vi "Gyro Angle.vi"() -> (13 "Angle":dbl)   [LabVIEW 2014]
uses:
  Global Variables/Refnum Names.vi
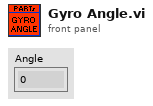
[diagram p1: front panel]
types:
  T1 = typedef "WPI_GyroDevRef.ctl" = cluster{"DevStatus":errorcluster, "Analog Module":T2, "Analog Channel":T3, "Offset":dbl, "Gain (VoltsPerDegree/Second)":dbl}
  T2 = typedef "FPGA_TypedefAnalogModule.ctl" = enum16{"Controller 1"}
  T3 = typedef "FPGA_AIChannel.ctl" = enum8{"AI 0", "AI 1", "AI 2", "AI 3", "AI MXP 0", "AI MXP 1", "AI MXP 2", "AI MXP 3", "Invalid"}
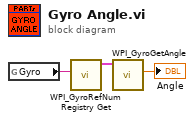
[diagram p0: block diagram]
diagram:
  n1 = global read "Refnum Names.vi" "Gyro"() -> (w2:string)
  n2 = call <vilib>:"WPI_GyroRefNum Registry Get.vi"("refnum name"=w2) -> ("GyroDevRef"=w1:T1)  [unwired: 9 in, 1 out]
  n3 = call <vilib>:"WPI_GyroGetAngle.vi"("GyroDevRef"=w1) -> ("Angle"=→"Angle":dbl)  [unwired: 7 in, 3 out]
